vi "GUI_HTU_VisaDiagnostics.vi"() -> ()   [LabVIEW 2013]
uses:
  Shared/GUI_Template/GUI_master/tcp_new_data_event.ctl
  Shared/GUI_Template/GUI_master/tcp new data cluster.ctl
  <vilib>/Utility/file.llb/Read From Spreadsheet File (DBL).vi
panel:
  out "data::4":dbl caption="Energy (nJ)" min=0.0 max=300000000.0 format="%.3f"
  in  "GUIdevice 4":string="U_FEL_EnergyMeter"
  in  "GUIdevice 3":string="U_VisaPlungers"
  in  "DigitalOutput.Channel 4::3":enum16{"on", "off"}(ring) caption="VISA e-beam 4"
  in  "DigitalOutput.Channel 2::3":enum16{"on", "off"}(ring) caption="VISA e-beam 6"
  in  "DigitalOutput.Channel 0::3":enum16{"on", "off"}(ring) caption="VISA e-beam 8"
  in  "DigitalOutput.Channel 7::3":enum16{"on", "off"}(ring) caption="VISA e-beam 1"
  in  "DigitalOutput.Channel 6::3":enum16{"on", "off"}(ring) caption="VISA e-beam 2"
  in  "DigitalOutput.Channel 5::3":enum16{"on", "off"}(ring) caption="VISA e-beam 3"
  in  "DigitalOutput.Channel 1::3":enum16{"on", "off"}(ring) caption="VISA e-beam 7"
  in  "DigitalOutput.Channel 3::3":enum16{"on", "off"}(ring) caption="VISA e-beam 5"
  in  "DigitalOutput.Channel 7::2":enum16{"on", "off"}(ring) caption="VISA e-beam 9"
  in  "GUIdevice 2":string="U_Valve_Daq"
  in  "Position::1":dbl caption="Current position" min=-1.0 max=4100.0 format="%.3f"
  out "Set Position":dbl
  in  "Eenrgy 9":bool
  in  "Eenrgy 8":bool
  in  "Eenrgy 7":bool
  in  "Eenrgy 6":bool
  in  "Eenrgy 5":bool
  in  "Eenrgy 4":bool
  in  "Eenrgy 3":bool
  in  "Eenrgy 2":bool
  in  "Eenrgy 1":bool
  in  "Spec 9":bool
  in  "Spec 8":bool
  in  "Spec 7":bool
  in  "Spec 6":bool
  in  "Spec 5":bool
  in  "Spec 4":bool
  in  "Spec 3":bool
  in  "Spec 2":bool
  in  "Spec 1":bool
  in  "Mode 9":bool
  in  "Mode 8":bool
  in  "Mode 7":bool
  in  "Mode 6":bool
  in  "Mode 5":bool
  in  "Mode 4":bool
  in  "Mode 3":bool
  in  "Mode 2":bool
  out "config":dbl[][](array[numeric]) format="%0.3f"
  in  "Mode 1":bool
  in  "M":bool caption="Blank Button"
  in  "UDP error message":string
  in  "GUIdevice 1":string="U_Velmex"
  out "error IO 2":errorcluster
  out "tcp data event":T1
  in  "stop":bool
  # "HTU Visa diagnostics"
  # "Visa1\nEMQ1"
  # "Visa2\nEMQ2"
  # "Visa3"
  # "Visa4\nEMQ1"
  # "Visa5\nEMQ2"
  # "Visa6"
  # "Visa7\nEMQ1"
  # "Visa8\nEMQ2"
  # "Visa9"
  # "Plunger"
  # "Mode Cam"
  # "Spectrometer"
  # "Energy meter"
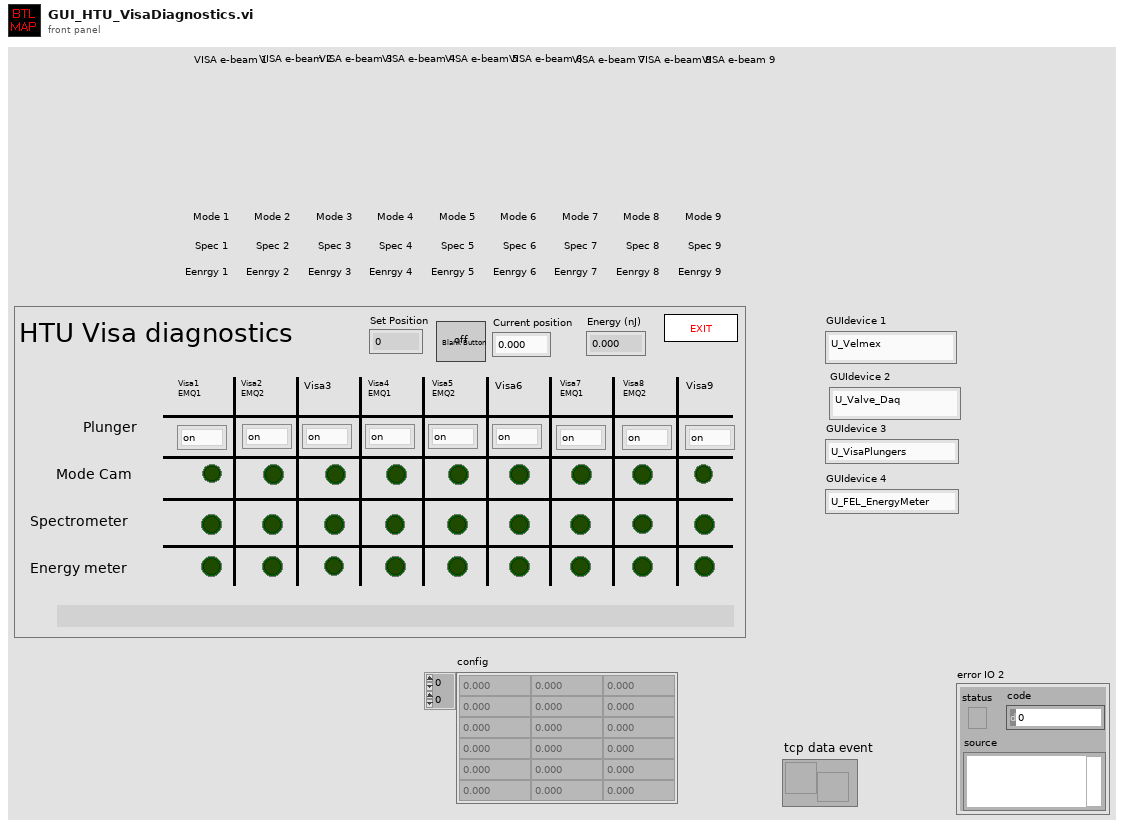
[diagram p1: front panel]
types:
  T1 = typedef "tcp_new_data_event.ctl" = refnum<user-event>
  T2 = typedef "tcp new data cluster.ctl" = cluster{"EventEnum":enum16{"new data", "connection status update"}, "Device name":string}
  T3 = enum32{"invalid app kind", "Development System", "Run Time System", "Student Edition", "Embedded LabVIEW", "Evaluation", "Custom"}
  T4 = enum32{"Invalid", "Standard", "Closed", "Hidden", "Minimized", "Maximized"}
  T5 = cluster{"Core":cluster{"Current VI Reference":refnum<vi>, "Close Panel on Exit?":bool}, "Row":i32, "Col":i32, "setPosition":dbl}
  T6 = cluster{"Current VI Reference":refnum<vi>, "Close Panel on Exit?":bool}
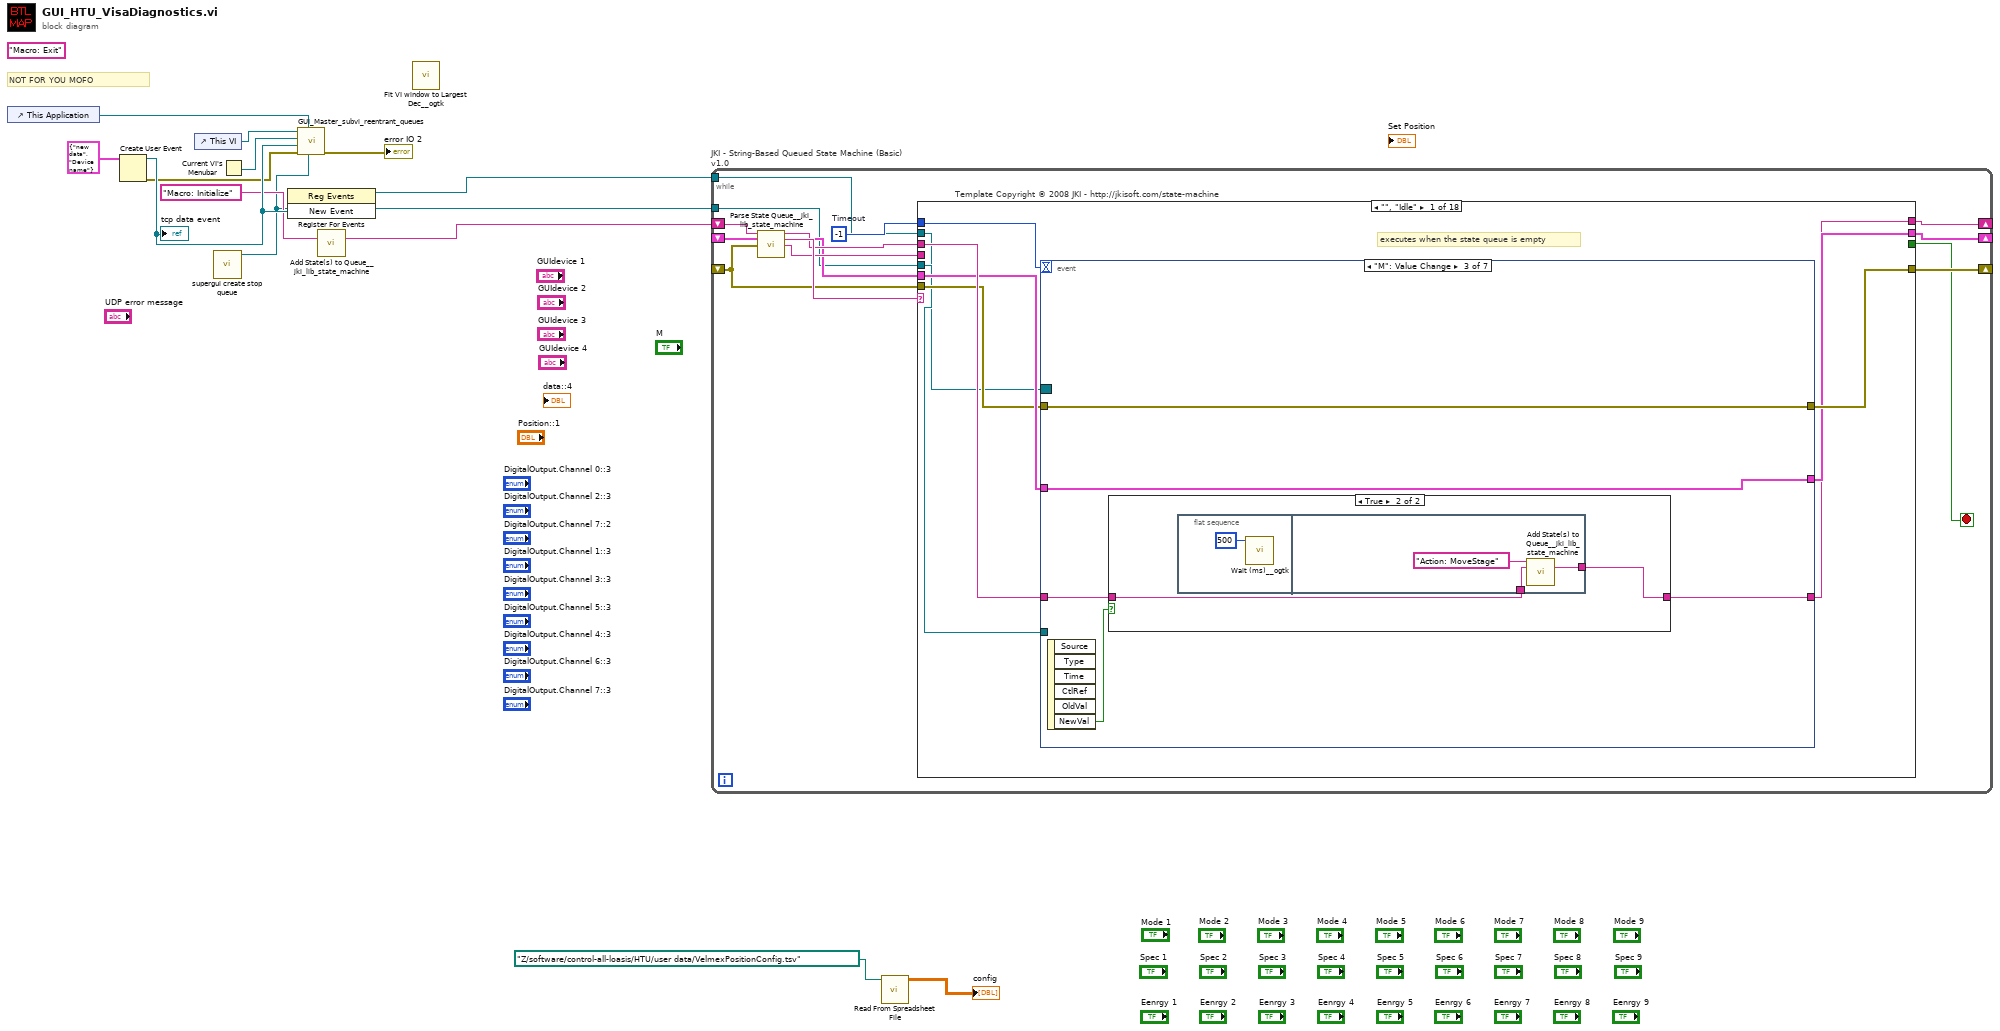
[diagram p0: block diagram]
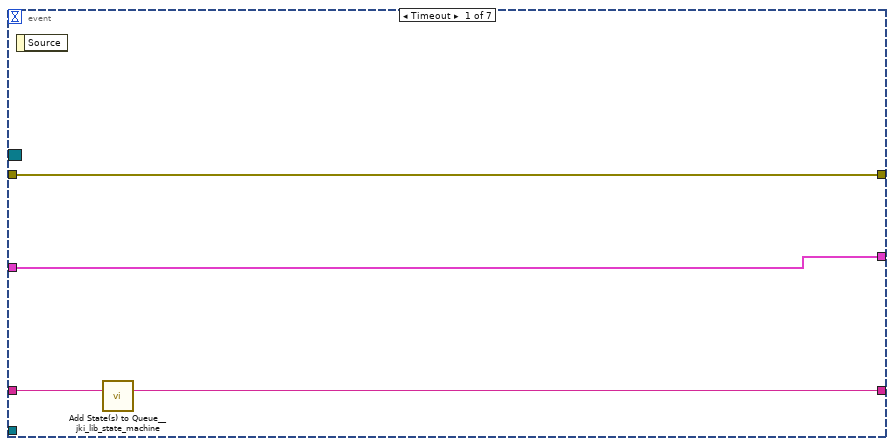
[diagram p2: hidden frame]
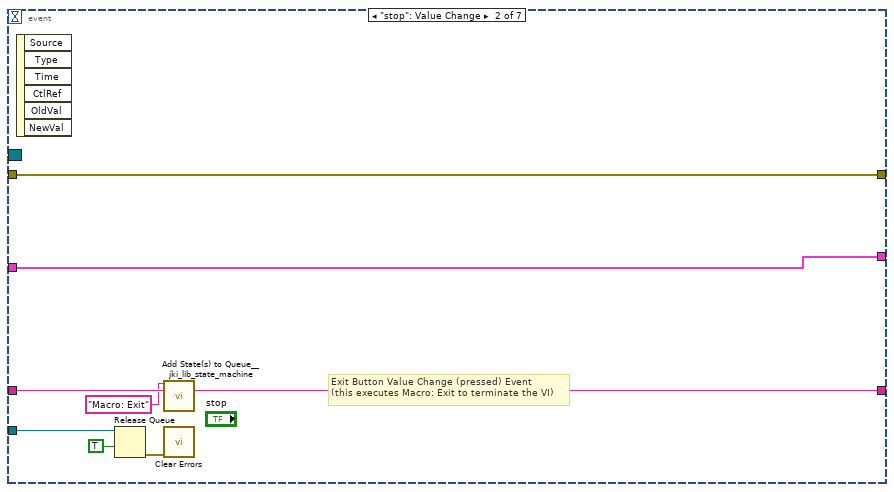
[diagram p3: hidden frame]
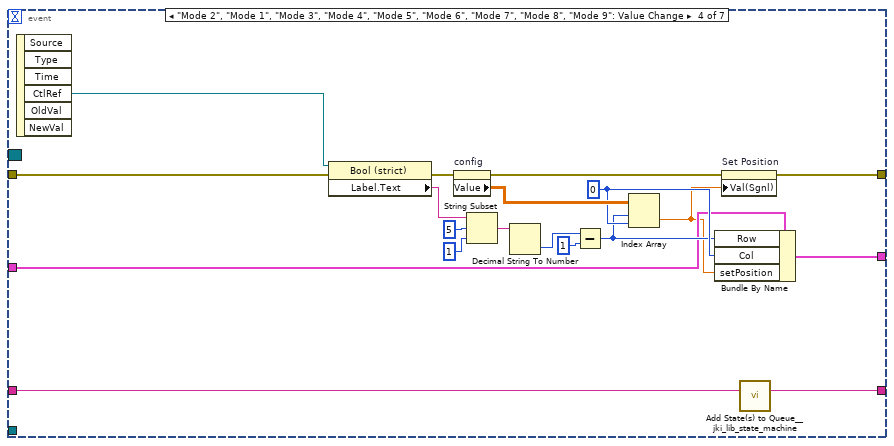
[diagram p5: hidden frame]
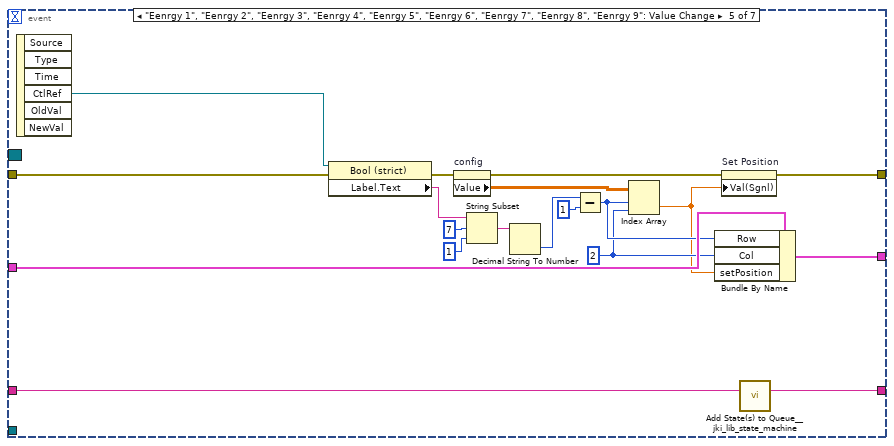
[diagram p6: hidden frame]
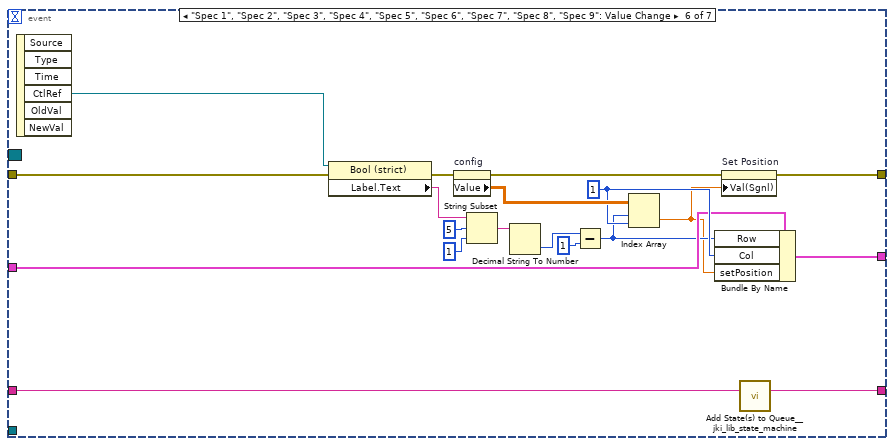
[diagram p7: hidden frame]
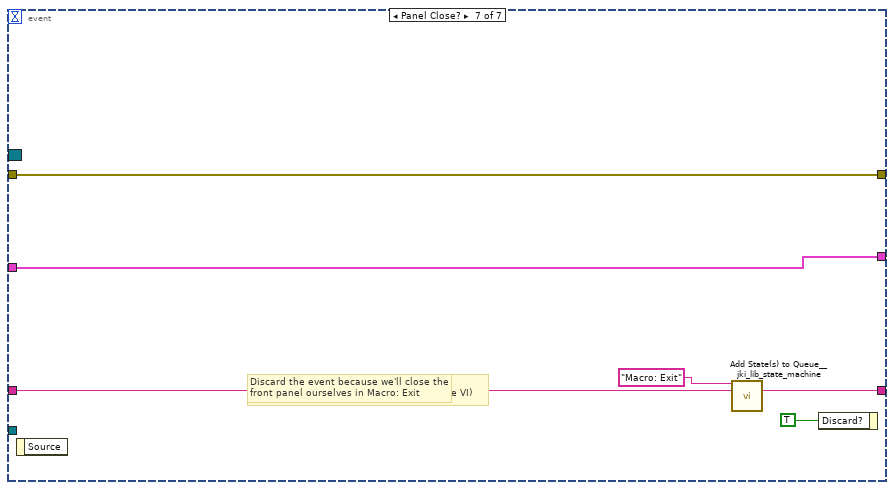
[diagram p8: hidden frame]
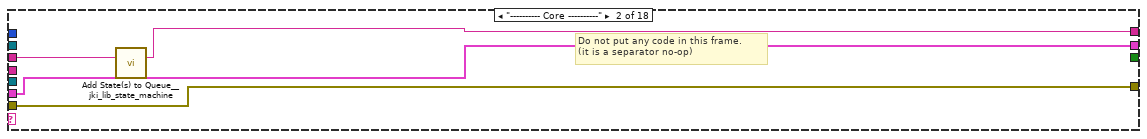
[diagram p9: hidden frame]
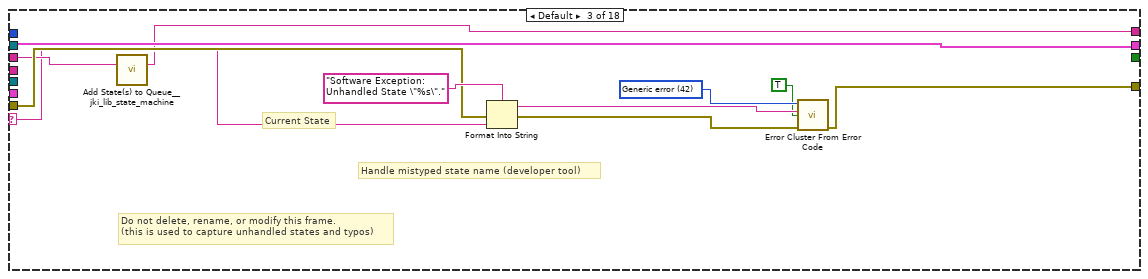
[diagram p10: hidden frame]
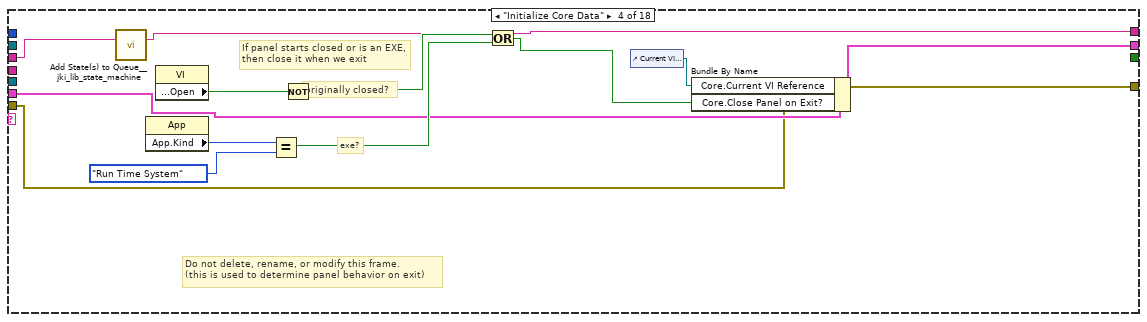
[diagram p11: hidden frame]
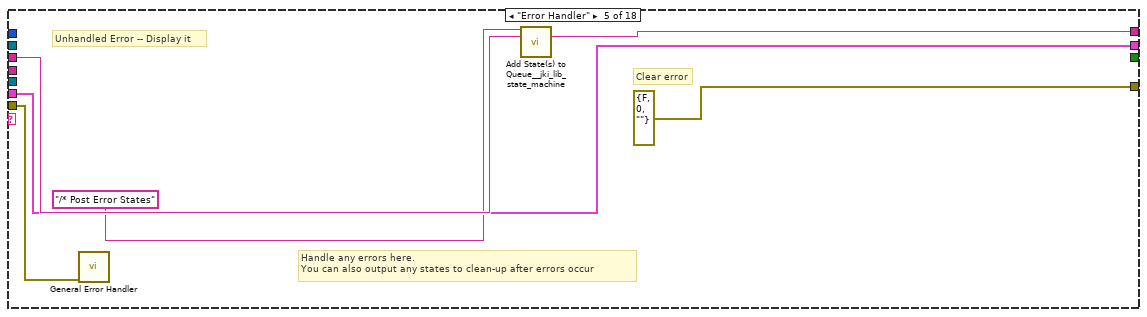
[diagram p12: hidden frame]
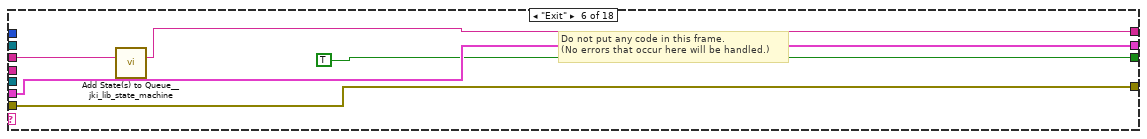
[diagram p13: hidden frame]
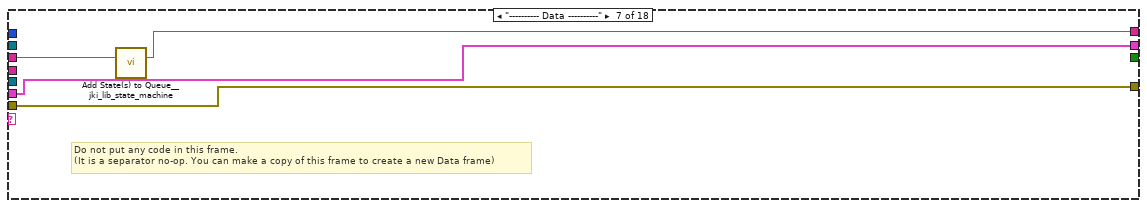
[diagram p14: hidden frame]
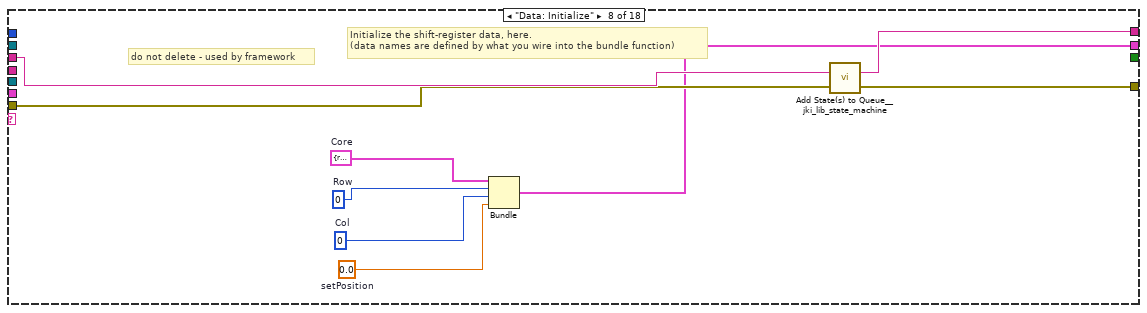
[diagram p15: hidden frame]
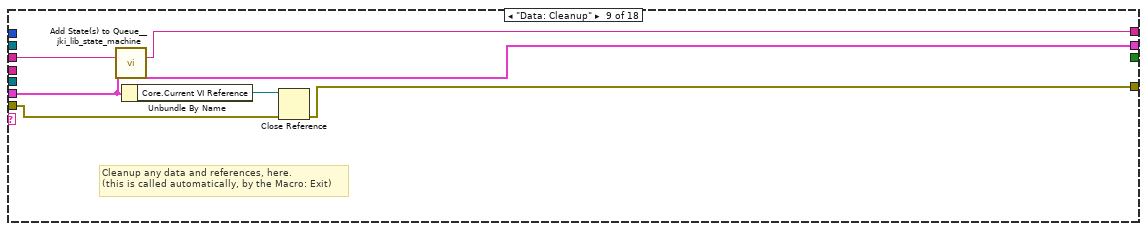
[diagram p16: hidden frame]
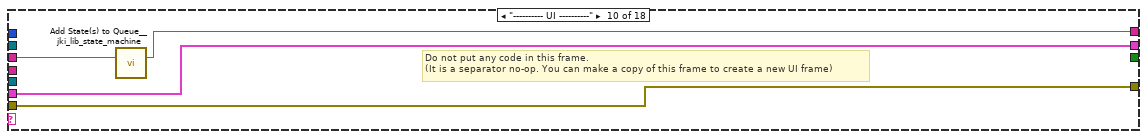
[diagram p17: hidden frame]
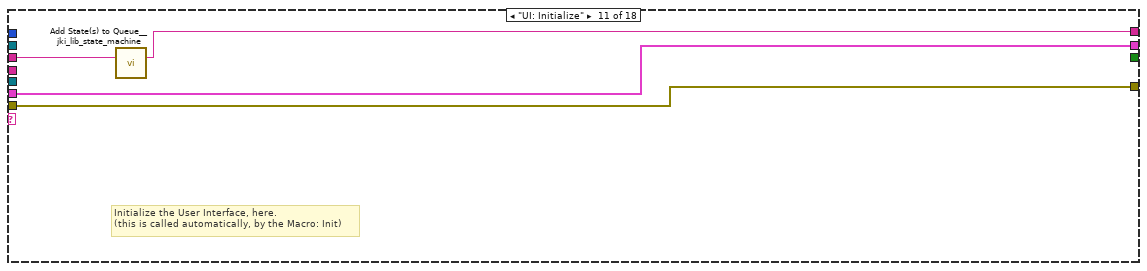
[diagram p18: hidden frame]
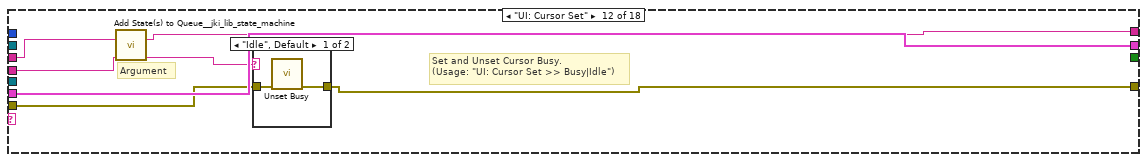
[diagram p19: hidden frame]
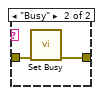
[diagram p20: hidden frame]
diagram:
  (unwired) "Macro: Exit"
  # "NOT FOR YOU MOFO"
  n1 = control-ref of="This Application"() -> (w13:refnum<vi>)
  n2 = Create User Event(user event datatype=T2 {"EventEnum"=enum."new data", "Device name"="Device name"} ("New Event")) -> (user event=w12:refnum<user-event>, error out=w11:errorcluster)  [unwired: 1 in]
  "tcp data event" <- w12
  n3 = control-ref of="This VI"() -> (w7:refnum<vi>)
  n4 = call "supergui create stop queue.vi"() -> ("STOP Queue out"=w3:refnum<queue>)  [unwired: 11 in]
  n5 = Current VI's Menubar() -> (w9:refnum<k9>)
  n6 = register-events(w12) -> (reference out=w4:refnum<event-registration>)  [unwired: 2 in, 1 out]
  n7 = call "GUI_Master_subvi_reentrant_queues.vi"("STOP Queue in"=w3, "This Application"=w13, "error in (no error)"=w11, "tcp data event"=w12, "Caller menu reference"=w9, "Caller VI ref"=w7) -> ("error out"=→"error IO 2":errorcluster)  [unwired: 5 in]
  n8 = call <vilib>:"Add State(s) to Queue__jki_lib_state_machine.vi"("State(s) in (\"\")"="Macro: Initialize") -> ("States Out"=w5:string)  [unwired: 14 in]
  n9 = call <userlib>:"Fit VI window to Largest Dec__ogtk.vi"() -> ()  [unwired: 6 in, 2 out]
  n10 = while "JKI - String-Based Queued State Machine (Basic) v1.0" {
    shift-right: [w20] -> _
    shift-left: _ -> [w19]
    shift-right: [w22] -> _
    shift-left: _ -> [w17]
    shift-right: [w14] -> _
    shift-left: w5 -> [w23]
    tunnel: w4 -> [w16]
    tunnel: w3 -> [w15]
    stop <- w21 stop-if-true
    w18 = -1  # Timeout
    # "Template Copyright © 2008 JKI - http://jkisoft.com/state-machine"
    n11 = call <vilib>:"Parse State Queue__jki_lib_state_machine.vi"("State Queue"=w23, "Error In (no error)"=w17) -> ("Remaining States"=w25:string, "Current State"=w26:string, "Arguments"=w24:string)  [unwired: 11 in]
    n12 = case shown="\"\", \"Idle\"" w26 {
      selector: w26 -> [_ _ w128 _ _ _ _ _ _ _ _ _ _ _ _ _ _ _]
      tunnel: w25 -> [w35 w126 w131 w149 w155 w160 w164 w172 w178 w182 w186 w192 w203 w229 w234 w244 w248 w254]
      tunnel: w24 -> [_ _ _ _ _ _ _ _ _ _ _ w188 w199 _ _ _ _ _]
      tunnel: w19 -> [w34 w124 w130 w141 w154 w159 w162 _ w174 w180 w185 w191 w198 w227 w232 w236 w246 w252]
      tunnel: [w33 w125 w133 w138 errorcluster {"status"=FALSE, "code"=0, "source"=""} ("error out") w158 w163 w171 w176 w181 w184 w189 w201 w228 w233 w243 w247 w249] -> w22
      tunnel: w17 -> [w32 w125 w132 w138 w153 w158 w163 w171 w177 w181 w184 w190 w202 w228 w233 w243 w247 w250]
      tunnel: [_ _ _ _ _ TRUE _ _ _ _ _ _ _ _ _ _ _ _] -> w21
      tunnel: [w29 w124 w130 w140 w154 w159 w162 w168 w174 w180 w185 w191 w198 w227 w232 w236 w246 w252] -> w20
      tunnel: w18 -> [w31 _ _ _ _ _ _ _ _ _ _ _ _ _ _ _ _ _]
      tunnel: w16 -> [w27 _ _ _ _ _ _ _ _ _ _ _ _ _ _ _ _ _]
      tunnel: w15 -> [w30 _ _ _ _ _ _ _ _ _ _ _ _ _ _ _ _ _]
      tunnel: [w28 w123 w127 w139 w150 w156 w161 w169 w173 w179 w183 w187 w197 w226 w230 w235 w245 w253] -> w14
      frame "", "Idle" {
        # "executes when the state queue is empty"
        n13 = event shown="[2] \"M\": Value Change" {
          selector: w27 -> [_ _ _ _ _ _ _]
          dyn-events: _ -> [_ _ _ _ _ _ _]
          timeout: w31 -> [_ _ _ _ _ _ _]
          tunnel: w35 -> [w39 w47 w50 w78 w97 w116 w122]
          tunnel: [w38 w46 w49 w77 w96 w115 w121] -> w28
          tunnel: w34 -> [w36 w44 w48 w66 w90 w105 w119]
          tunnel: [w37 w45 w52 w60 w79 w98 w120] -> w33
          tunnel: w32 -> [w37 w45 w52 w64 w83 w102 w120]
          tunnel: [w36 w44 w48 w65 w89 w104 w119] -> w29
          tunnel: w30 -> [_ w41 _ _ _ _ _]
          event Timeout {
            n14 = event-data() -> ()  [unwired: 1 in, 1 out]
            n15 = call <vilib>:"Add State(s) to Queue__jki_lib_state_machine.vi"("State(s) in (\"\")"=w39) -> ("States Out"=w38:string)  [unwired: 14 in]
          }
          event "stop": Value Change {
            # "Exit Button Value Change (pressed) Event\n(this executes Macro: Exit to terminate the VI)"
            n16 = event-data() -> ()  [unwired: 1 in, 6 out]
            n17 = Release Queue(queue=w41, force destroy? (F)=TRUE) -> (error out=w42:errorcluster)  [unwired: 1 in, 2 out]
            n18 = call <vilib>:"Add State(s) to Queue__jki_lib_state_machine.vi"("State(s) in Front (\"\")"="Macro: Exit", "State(s) in (\"\")"=w47) -> ("States Out"=w46:string)  [unwired: 13 in]
            n19 = call <vilib>:"Clear Errors.vi"("error in (no error)"=w42) -> ()  [unwired: 6 in, 1 out]
          }
          event "M": Value Change {
            n20 = event-data() -> ("NewVal"=w51:bool)  [unwired: 1 in, 5 out]
            n21 = case shown="True" w51 {
              tunnel: w50 -> [w53 w55]
              tunnel: [w53 w54] -> w49
              frame False {
              }
              frame True {
                n22 = flat-sequence {
                  tunnel: w55 -> [w58]
                  tunnel: [w57] -> w54
                  frame #0 {
                    n23 = call <userlib>:"Wait (ms)__ogtk.vi"("milliseconds to wait"=u32 500) -> ()  [unwired: 9 in, 2 out]
                  }
                  frame #1 {
                    n24 = call <vilib>:"Add State(s) to Queue__jki_lib_state_machine.vi"("State(s) in Front (\"\")"="Action: MoveStage" ("State(s) in Front (\"\")"), "State(s) in (\"\")"=w58) -> ("States Out"=w57:string)  [unwired: 13 in]
                  }
                }
              }
            }
          }
          event "Mode 2", "Mode 1", "Mode 3", "Mode 4", "Mode 5", "Mode 6", "Mode 7", "Mode 8", "Mode 9": Value Change {
            w68 = 0 ("Col")
            n25 = event-data() -> ("CtlRef"=w76:refnum<vi>)  [unwired: 1 in, 5 out]
            n26 = property class="Bool (strict)"(reference=w76, error in=w64) -> (error out=w63:errorcluster, "Label.Text"=w75:string)  [unwired: 1 out]
            n27 = property on="config" class="Arr (strict)"(error in=w63) -> (error out=w61:errorcluster, "Value"=w69:dbl[][])  [unwired: 1 in, 1 out]
            n28 = String Subset(string=w75, offset (0)=5, length (rest)=1 ("length (rest)")) -> (substring=w72:string)
            n29 = Decimal String To Number(string=w72) -> (number=w71:i32)  [unwired: 2 in, 1 out]
            n30 = Subtract(x=w71, y=1) -> (x-y=w67:i32)
            n31 = Index Array(array=w69, index (row)=w67, index (col)=w68) -> (element=w62:dbl)
            n32 = Bundle By Name(cluster=w66, "Row"=w67, "Col"=w68, "setPosition"=w62) -> (w65:T5)
            n33 = property on="Set Position" class="DigNum (strict)"(error in=w61, "Val(Sgnl)"=w62) -> (error out=w60:errorcluster)  [unwired: 1 in, 1 out]
            n34 = call <vilib>:"Add State(s) to Queue__jki_lib_state_machine.vi"("State(s) in (\"\")"=w78) -> ("States Out"=w77:string)  [unwired: 14 in]
          }
          event "Eenrgy 1", "Eenrgy 2", "Eenrgy 3", "Eenrgy 4", "Eenrgy 5", "Eenrgy 6", "Eenrgy 7", "Eenrgy 8", "Eenrgy 9": Value Change {
            w84 = 2 ("Col")
            n35 = event-data() -> ("CtlRef"=w95:refnum<vi>)  [unwired: 1 in, 5 out]
            n36 = property class="Bool (strict)"(reference=w95, error in=w83) -> (error out=w82:errorcluster, "Label.Text"=w94:string)  [unwired: 1 out]
            n37 = property on="config" class="Arr (strict)"(error in=w82) -> (error out=w81:errorcluster, "Value"=w86:dbl[][])  [unwired: 1 in, 1 out]
            n38 = String Subset(string=w94, offset (0)=7, length (rest)=1 ("length (rest)")) -> (substring=w91:string)
            n39 = Decimal String To Number(string=w91) -> (number=w88:i32)  [unwired: 2 in, 1 out]
            n40 = Subtract(x=w88, y=1) -> (x-y=w85:i32)
            n41 = Index Array(array=w86, index (row)=w85, index (col)=w84) -> (element=w80:dbl)
            n42 = Bundle By Name(cluster=w90, "Row"=w85, "Col"=w84, "setPosition"=w80) -> (w89:T5)
            n43 = property on="Set Position" class="DigNum (strict)"(error in=w81, "Val(Sgnl)"=w80) -> (error out=w79:errorcluster)  [unwired: 1 in, 1 out]
            n44 = call <vilib>:"Add State(s) to Queue__jki_lib_state_machine.vi"("State(s) in (\"\")"=w97) -> ("States Out"=w96:string)  [unwired: 14 in]
          }
          event "Spec 1", "Spec 2", "Spec 3", "Spec 4", "Spec 5", "Spec 6", "Spec 7", "Spec 8", "Spec 9": Value Change {
            w106 = 1 ("Col")
            n45 = event-data() -> ("CtlRef"=w114:refnum<vi>)  [unwired: 1 in, 5 out]
            n46 = property class="Bool (strict)"(reference=w114, error in=w102) -> (error out=w101:errorcluster, "Label.Text"=w113:string)  [unwired: 1 out]
            n47 = property on="config" class="Arr (strict)"(error in=w101) -> (error out=w99:errorcluster, "Value"=w107:dbl[][])  [unwired: 1 in, 1 out]
            n48 = String Subset(string=w113, offset (0)=5, length (rest)=1 ("length (rest)")) -> (substring=w110:string)
            n49 = Decimal String To Number(string=w110) -> (number=w109:i32)  [unwired: 2 in, 1 out]
            n50 = Subtract(x=w109, y=1) -> (x-y=w103:i32)
            n51 = Index Array(array=w107, index (row)=w103, index (col)=w106) -> (element=w100:dbl)
            n52 = Bundle By Name(cluster=w105, "Row"=w103, "Col"=w106, "setPosition"=w100) -> (w104:T5)
            n53 = property on="Set Position" class="DigNum (strict)"(error in=w99, "Val(Sgnl)"=w100) -> (error out=w98:errorcluster)  [unwired: 1 in, 1 out]
            n54 = call <vilib>:"Add State(s) to Queue__jki_lib_state_machine.vi"("State(s) in (\"\")"=w116) -> ("States Out"=w115:string)  [unwired: 14 in]
          }
          event Panel Close? {
            # "Discard the event because we'll close the front panel ourselves in Macro: Exit"
            # "Close Panel button (pressed) Event\n(this executes Macro: Exit to terminate the VI)"
            n55 = event-data() -> ()  [unwired: 1 in, 1 out]
            n56 = call <vilib>:"Add State(s) to Queue__jki_lib_state_machine.vi"("State(s) in Front (\"\")"="Macro: Exit", "State(s) in (\"\")"=w122) -> ("States Out"=w121:string)  [unwired: 13 in]
            n57 = event-data("Discard?"=TRUE) -> ()  [unwired: 1 in, 1 out]
          }
        }
      }
      frame "---------- Core ----------" {
        # "Do not put any code in this frame.\n(it is a separator no-op)"
        n58 = call <vilib>:"Add State(s) to Queue__jki_lib_state_machine.vi"("State(s) in (\"\")"=w126) -> ("States Out"=w123:string)  [unwired: 14 in]
      }
      frame Default {
        w136 = 42 items=["No error", "Argument error", "Memory is full", "Out of zone", "End of file", "File already open", "Generic file I/O error", "File not found", "File permission error", "Disk is full", "Duplicate path", "Too many files open", "System feature not enabled", "Resource file not found", "Cannot add resource", "Resource not found", "Image not found", "Image memory error", "Pen does not exist", "Config type invalid", "Config token not found", "Config parse error", "Config memory error", "Bad external code format", "Bad external code offset", "External code not present", "Null window", "Destroy window error", "Null menu", "Print aborted", "Bad print record", "Print driver error", "Windows error during printing", "Memory error during printing", "Print dialog error", "Generic print error", "Invalid device refnum", "Device not found", "Device parameter error", "Device unit error", "Cannot open device", "Device call aborted", "Generic error", "Cancelled by user", "Object ID too low", "Object ID too high", "Object not in heap", "Unknown heap", "Unknown object (invalid DefProc)", "Unknown object (DefProc not in table)", "Message out of range", "Invalid (null) method", "Unknown message", "Manager call not supported", "Bad address", "Network operation in progress", "Network operation timed out", "Connection is busy", "Network attribute not supported", "Network error", "Address in use", "System out of memory", "Connection aborted", "Connection refused", "Not connected", "Already connected", "Connection closed", "Initialization error (interapplication manager)", "Bad occurrence", "Wait on unbound occurrence handler", "Occurrence queue overflow", "Datalog type conflict", "Unused", "Unrecognized type (interapplication manager)", "Memory corrupt", "Failed to make temporary DLL", "Old CIN version", "Drag socket not found", "Failed to load drop-object", "Failed to register OLE object", "Failed to release OLE object", "Format specifier type mismatch", "Unknown format specifier", "Too few format specifiers", "Too many format specifiers", "Scan failed", "Newer CIN version", "Error converting to variant", "Runtime menu error", "Password tampered", "Variant attribute not found", "Incompatible variant data type", "Event data is not available", "Event Store is not present", "Occurrence is not found", "Event Queue is not created", "Event info is not available", "Refnum passed is NULL", "Error retrieving Class GUID", "Error retrieving CoClass GUID", "Error retrieving TypeLib GUID.", "Bad built application magic bytes.", "Specific driver is different from the specific driver associated with the Logical Name.", "There is no session opened to the class driver.", "Max Error", "MAX - Error with config objects", "MAX - Error loading configuration", "MAX - Group not supported"]
        # "Current State"
        # "Do not delete, rename, or modify this frame.\n(this is used to capture unhandled states and typos)"
        # "Handle mistyped state name (developer tool)"
        n59 = call <vilib>:"Add State(s) to Queue__jki_lib_state_machine.vi"("State(s) in (\"\")"=w131) -> ("States Out"=w127:string)  [unwired: 14 in]
        n60 = Format Into String(format string="Software Exception: Unhandled State \"%s\"." ("message"), error in=w132, w128) -> (resulting string=w135:string, error out=w134:errorcluster)  [unwired: 1 in]
        n61 = call <vilib>:"Error Cluster From Error Code.vi"("show call chain? (False)"=TRUE, "error in (no error)"=w134, "error message (\"\")"=w135, "error code (0)"=w136) -> ("error out"=w133:errorcluster)  [unwired: 5 in]
      }
      frame "Initialize Core Data" {
        # "Do not delete, rename, or modify this frame.\n(this is used to determine panel behavior on exit)"
        # "originally closed?"
        # "exe?"
        # "If panel starts closed or is an EXE, then close it when we exit"
        n62 = call <vilib>:"Add State(s) to Queue__jki_lib_state_machine.vi"("State(s) in (\"\")"=w149) -> ("States Out"=w139:string)  [unwired: 14 in]
        n63 = property class="App"() -> ("App.Kind"=w147:T3)  [unwired: 2 in, 2 out]
        n64 = property class="VI"() -> ("Front Panel.Open"=w148:bool)  [unwired: 2 in, 2 out]
        n65 = Equal?(x=w147, y=T3."Run Time System" ("Application:Kind")) -> (x = y?=w144:bool)
        n66 = Not(x=w148) -> (.not. x?=w145:bool)
        n67 = Or(x=w145, y=w144) -> (x .or. y?=w143:bool)
        n68 = control-ref of="Current VI Reference"() -> (w142:refnum<vi>)
        n69 = Bundle By Name(cluster=w141, "Core.Current VI Reference"=w142, "Core.Close Panel on Exit?"=w143) -> (w140:T5)
      }
      frame "Error Handler" {
        # "Unhandled Error -- Display it"
        # "Handle any errors here.\nYou can also output any states to clean-up after errors occur"
        # "Clear error"
        n70 = call <vilib>:"General Error Handler.vi"("error in (no error)"=w153) -> ()  [unwired: 10 in, 5 out]
        n71 = call <vilib>:"Add State(s) to Queue__jki_lib_state_machine.vi"("State(s) in Front (\"\")"="/* Post Error States", "State(s) in (\"\")"=w155) -> ("States Out"=w150:string)  [unwired: 13 in]
      }
      frame "Exit" {
        # "Do not put any code in this frame.\n(No errors that occur here will be handled.)"
        n72 = call <vilib>:"Add State(s) to Queue__jki_lib_state_machine.vi"("State(s) in (\"\")"=w160) -> ("States Out"=w156:string)  [unwired: 14 in]
      }
      frame "---------- Data ----------" {
        # "Do not put any code in this frame.\n(It is a separator no-op. You can make a copy of this frame to create a new Data frame)"
        n73 = call <vilib>:"Add State(s) to Queue__jki_lib_state_machine.vi"("State(s) in (\"\")"=w164) -> ("States Out"=w161:string)  [unwired: 14 in]
      }
      frame "Data: Initialize" {
        w165 = 0.0  # setPosition
        w166 = 0  # Col
        w167 = 0  # Row
        w170 = T6 {"Current VI Reference"=refnum, "Close Panel on Exit?"=FALSE}  # Core
        # "do not delete - used by framework"
        # "Initialize the shift-register data, here.\n(data names are defined by what you wire into the bundle function)"
        n74 = Bundle("Core"=w170, "Row"=w167, "Col"=w166, "setPosition"=w165) -> (w168:T5)  [unwired: 1 in]
        n75 = call <vilib>:"Add State(s) to Queue__jki_lib_state_machine.vi"("State(s) in (\"\")"=w172) -> ("States Out"=w169:string)  [unwired: 14 in]
      }
      frame "Data: Cleanup" {
        # "Cleanup any data and references, here.\n(this is called automatically, by the Macro: Exit)"
        n76 = call <vilib>:"Add State(s) to Queue__jki_lib_state_machine.vi"("State(s) in (\"\")"=w178) -> ("States Out"=w173:string)  [unwired: 14 in]
        n77 = Unbundle By Name(w174) -> ("Core.Current VI Reference"=w175:refnum<vi>)
        n78 = Close Reference(reference=w175, error in (no error)=w177) -> (error out=w176:errorcluster)
      }
      frame "---------- UI ----------" {
        # "Do not put any code in this frame.\n(It is a separator no-op. You can make a copy of this frame to create a new UI frame)"
        n79 = call <vilib>:"Add State(s) to Queue__jki_lib_state_machine.vi"("State(s) in (\"\")"=w182) -> ("States Out"=w179:string)  [unwired: 14 in]
      }
      frame "UI: Initialize" {
        # "Initialize the User Interface, here.\n(this is called automatically, by the Macro: Init)"
        n80 = call <vilib>:"Add State(s) to Queue__jki_lib_state_machine.vi"("State(s) in (\"\")"=w186) -> ("States Out"=w183:string)  [unwired: 14 in]
      }
      frame "UI: Cursor Set" {
        # "Argument"
        # "Set and Unset Cursor Busy.\n(Usage: \"UI: Cursor Set >> Busy|Idle\")"
        n81 = call <vilib>:"Add State(s) to Queue__jki_lib_state_machine.vi"("State(s) in (\"\")"=w192) -> ("States Out"=w187:string)  [unwired: 14 in]
        n82 = case shown="\"Idle\", Default" w188 {
          tunnel: w190 -> [w194 w196]
          tunnel: [w193 w195] -> w189
          frame "Idle", Default {
            n83 = call <vilib>:"Unset Busy.vi"("error in (no error)"=w194) -> ("error out"=w193:errorcluster)  [unwired: 10 in]
          }
          frame "Busy" {
            n84 = call <vilib>:"Set Busy.vi"("error in (no error)"=w196) -> ("error out"=w195:errorcluster)  [unwired: 9 in, 1 out]
          }
        }
      }
      frame "UI: Front Panel State" {
        # "Argument"
        # "Set Front Panel Open or Closed\n(Usage: \"UI: Front Panel State >> Open|Close\")"
        n85 = call <vilib>:"Add State(s) to Queue__jki_lib_state_machine.vi"("State(s) in (\"\")"=w203) -> ("States Out"=w197:string)  [unwired: 14 in]
        n86 = Unbundle By Name(w198) -> ("Core.Current VI Reference"=w200:refnum<vi>)
        n87 = case shown="\"Open\", Default" w199 {
          tunnel: w202 -> [w208 w220]
          tunnel: [w209 w221] -> w201
          tunnel: w200 -> [w204 w216]
          frame "Open", Default {
            n88 = property class="VI"(reference=w204, error in=w208) -> (reference out=w206:refnum<vi>, error out=w207:errorcluster, "Front Panel.Open"=w205:bool)
            n89 = case shown="False" w205 {
              tunnel: [w212 w215] -> w209
              tunnel: w207 -> [w211 w215]
              tunnel: w206 -> [w210 _]
              frame False {
                n90 = invoke class="VI" method="FP.Open"(reference=w210, error in=w211, "Activate"=TRUE, "State"=T4."Standard") -> (error out=w212:errorcluster)  [unwired: 1 in, 4 out]
              }
              frame True {
              }
            }
          }
          frame "Close" {
            n91 = property class="VI"(reference=w216, error in=w220) -> (reference out=w218:refnum<vi>, error out=w219:errorcluster, "Front Panel.Open"=w217:bool)
            n92 = case shown="True" w217 {
              tunnel: [w222 w225] -> w221
              tunnel: w219 -> [w222 w224]
              tunnel: w218 -> [_ w223]
              frame False {
              }
              frame True {
                n93 = invoke class="VI" method="FP.Close"(reference=w223, error in=w224) -> (error out=w225:errorcluster)  [unwired: 1 in, 2 out]
              }
            }
          }
        }
      }
      frame "---------- Macro ----------" {
        # "Do not put any code in this frame.\n(It is a separator no-op. You can make a copy of this frame to create a new Macro frame)"
        n94 = call <vilib>:"Add State(s) to Queue__jki_lib_state_machine.vi"("State(s) in (\"\")"=w229) -> ("States Out"=w226:string)  [unwired: 14 in]
      }
      frame "Macro: Initialize" {
        w231 = "Data: Initialize\nInitialize Core Data\nUI: Initialize\nUI: Front Panel State >> Open"  # Data: Initialize Initialize Core Data UI: Initialize UI: Front Panel State >> Open
        # "Initialization Macro\n(This is called once, when the VI starts)"
        n95 = call <vilib>:"Add State(s) to Queue__jki_lib_state_machine.vi"("State(s) in Front (\"\")"=w231, "State(s) in (\"\")"=w234) -> ("States Out"=w230:string)  [unwired: 13 in]
      }
      frame "Macro: Exit" {
        # "Exit Macro\n(This is called once, when the VI exits)"
        n96 = Unbundle By Name(w236) -> ("Core.Close Panel on Exit?"=w237:bool)
        n97 = Select(t="UI: Front Panel State >> Close", s=w237, f="") -> (s? t:f=w240:string)
        n98 = call <vilib>:"Add State(s) to Queue__jki_lib_state_machine.vi"("State(s) in (\"\")"=w240, "State(s) at Back (\"\")"="Data: Cleanup\nExit") -> ("States Out"=w238:string)  [unwired: 13 in]
        n99 = call <vilib>:"Add State(s) to Queue__jki_lib_state_machine.vi"("State(s) in Front (\"\")"=w238, "State(s) in (\"\")"=w244) -> ("States Out"=w235:string)  [unwired: 13 in]
      }
      frame "---------- New Category ----------" {
        n100 = call <vilib>:"Add State(s) to Queue__jki_lib_state_machine.vi"("State(s) in (\"\")"=w248) -> ("States Out"=w245:string)  [unwired: 14 in]
      }
      frame "Action: MoveStage" {
        n101 = call <vilib>:"Add State(s) to Queue__jki_lib_state_machine.vi"("State(s) in (\"\")"=w254) -> ("States Out"=w253:string)  [unwired: 14 in]
        n102 = Unbundle By Name(w252) -> ("setPosition"=w251:dbl)
        n103 = property on="Position::1" class="DigNum (strict)"(error in=w250, "Val(Sgnl)"=w251) -> (error out=w249:errorcluster)  [unwired: 1 in, 1 out]
      }
    }
  }
  n104 = call-poly <vilib>:"Read From Spreadsheet File.vi"("file path (dialog if empty)"=path "Z:/software/control-all-loasis/HTU/user data/VelmexPositionConfig.tsv") -> ("all rows"=→"config":dbl[][])  [unwired: 6 in, 4 out]
